vi "Calculate Total Ramp Period.vi"(0 "Start Delay In":dbl[](array[numeric]), 2 "Default Ramp Rate":bool[](array[boolean]), 5 "Relative To":T1[](array[typedef]) items=["Power sequence start", "Previous source start", "Previous source end"], 7 "Level":dbl[](array[numeric]), 9 "Ramp Rate":dbl[](array[numeric]), 11 "Sequence Delta":dbl[](array[numeric])) -> (4 "Accumulative Start delays":dbl[](array[numeric]), 6 "Total Power Seq Period":dbl format="%#_6p", 8 "Rising Period":dbl[](array[numeric]) format="%#_6p", 10 "Max Sequence Period Index":i32)   [LabVIEW 2024, in "devicePowerSequencerCoreLogic.lvlib"]
uses:
  devicePowerSequencerCoreLogic.lvlib
  controls/Relative To.ctl
  Device Power Sequencer.lvlib
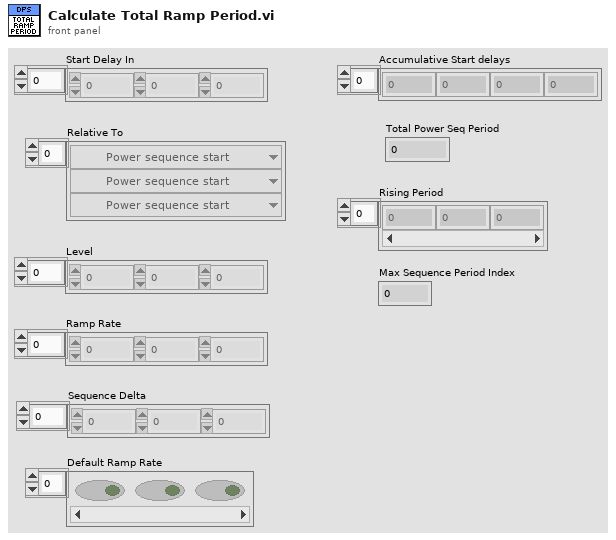
[diagram p1: front panel]
types:
  T1 = typedef "Device Power Sequencer.lvlib/Relative To.ctl" = u32
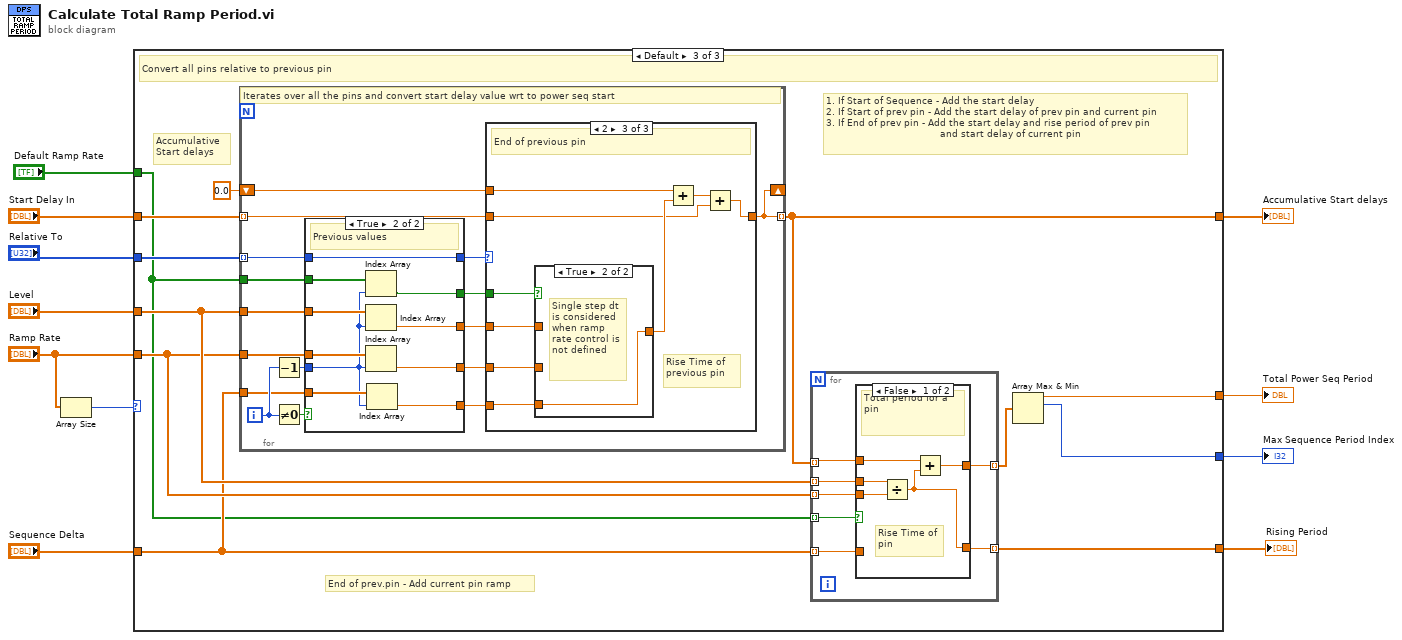
[diagram p0: block diagram]
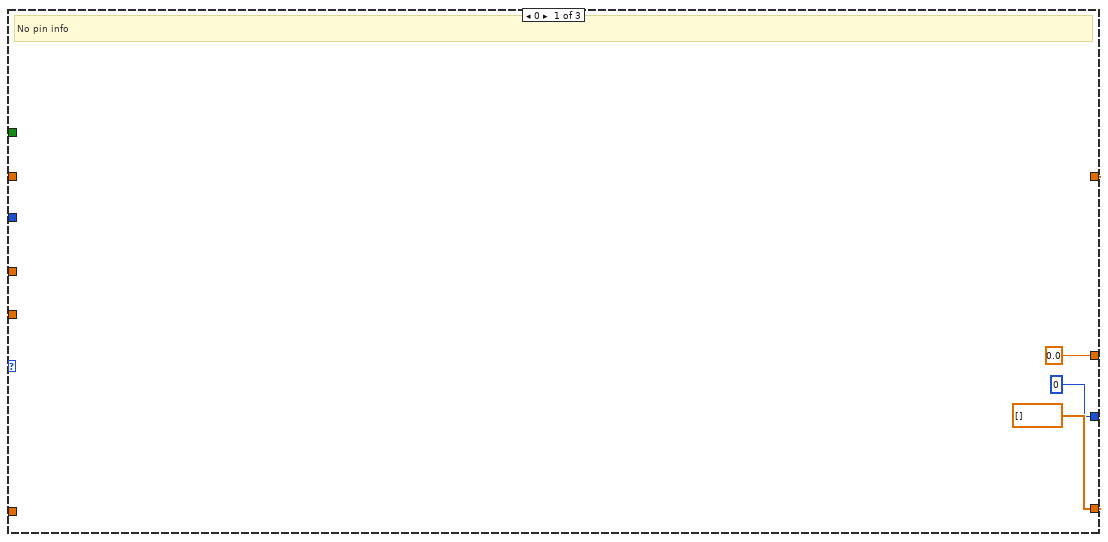
[diagram p2: hidden frame]
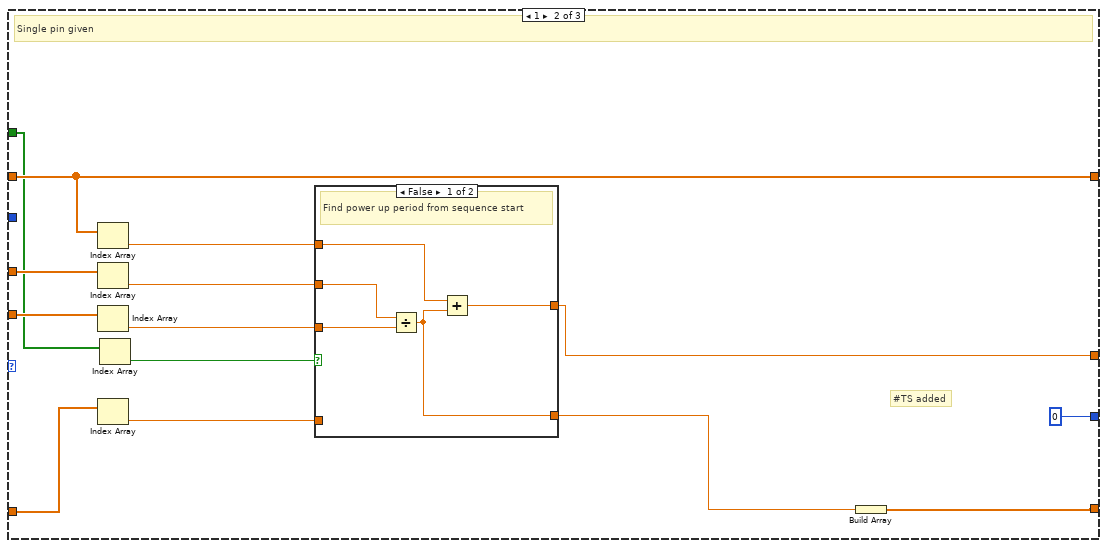
[diagram p3: hidden frame]
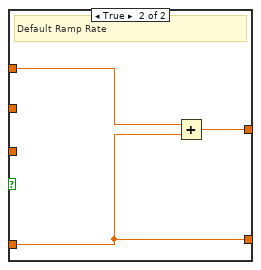
[diagram p4: hidden frame]
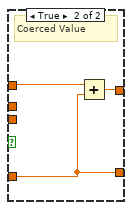
[diagram p5: hidden frame]
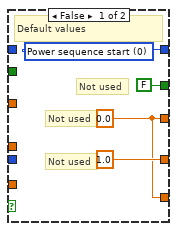
[diagram p6: hidden frame]
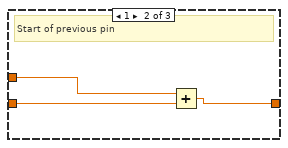
[diagram p8: hidden frame]
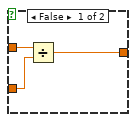
[diagram p9: hidden frame]
diagram:
  n1 = Array Size(array="Ramp Rate") -> (size(s)=w7:i32)
  n2 = case shown="Default" w7 {
    tunnel: "Start Delay In" -> [_ w21 w48]
    tunnel: "Relative To" -> [_ _ w47]
    tunnel: "Level" -> [_ w28 w45]
    tunnel: "Ramp Rate" -> [_ w27 w44]
    tunnel: [0.0 w20 w40] -> w9
    tunnel: [w14 w18 w39] -> w3
    tunnel: "Sequence Delta" -> [_ w23 w42]
    tunnel: [w14 w21 w41] -> w4
    tunnel: [0 0 w38] -> w2
    tunnel: "Default Ramp Rate" -> [_ w15 w37]
    frame 0 {
      w14 = dbl[] []
      # "No pin info"
    }
    frame 1 {
      # "#TS added"
      # "Single pin given"
      n3 = Index Array(array=w21) -> (element=w24:dbl)  [unwired: 1 in]
      n4 = Index Array(array=w28) -> (element=w25:dbl)  [unwired: 1 in]
      n5 = Index Array(array=w27) -> (element=w26:dbl)  [unwired: 1 in]
      n6 = Index Array(array=w23) -> (element=w22:dbl)  [unwired: 1 in]
      n7 = Index Array(array=w15) -> (element=w16:bool)  [unwired: 1 in]
      n8 = case shown="False" w16 {
        tunnel: [w33 w35] -> w20
        tunnel: w26 -> [w32 _]
        tunnel: w25 -> [w31 _]
        tunnel: w24 -> [w30 w36]
        tunnel: w22 -> [_ w34]
        tunnel: [w29 w34] -> w19
        frame False {
          # "Find power up period from sequence start"
          n9 = Divide(x=w31, y=w32) -> (x/y=w29:dbl)
          n10 = Add(x=w30, y=w29) -> (x+y=w33:dbl)
        }
        frame True {
          # "Default Ramp Rate"
          n11 = Add(x=w36, y=w34) -> (x+y=w35:dbl)
        }
      }
      n12 = Build Array(w19) -> (w18:dbl[])
    }
    frame Default {
      # "1. If Start of Sequence - Add the start delay\n2. If Start of prev pin - Add the start delay of prev pin and current pin\n3. If End of prev pin - Add the start delay and rise period of prev pin \n                                      and start delay of current pin"
      # "End of prev.pin - Add current pin ramp"
      # "Accumulative\nStart delays"
      # "Convert all pins relative to previous pin"
      n13 = for {
        tunnel: w48 -> [w79] mode=indexing
        tunnel: w47 -> [w67] mode=indexing
        tunnel: w44 -> [w75]
        tunnel: [w74] -> w41 mode=indexing
        shift-right: [w74] -> _
        shift-left: 0.0 ("Numeric") -> [w78]
        tunnel: w45 -> [w76]
        tunnel: w42 -> [w69]
        tunnel: w37 -> [w65]
        i -> [w73]
        # "Iterates over all the pins and convert start delay value wrt to power seq start"
        n14 = Decrement(x=w73) -> (x-1=w72:i32)
        n15 = Not Equal To 0?(x=w73) -> (x != 0?=w77:bool)
        n16 = case shown="True" w77 {
          tunnel: w76 -> [_ w93]
          tunnel: w75 -> [_ w92]
          tunnel: w72 -> [_ w85]
          tunnel: [w82 w91] -> w71
          tunnel: [1.0 ("Numeric") w90] -> w70
          tunnel: w69 -> [_ w89]
          tunnel: [w82 w88] -> w68
          tunnel: w67 -> [_ w87]
          tunnel: [w81 w87] -> w66
          tunnel: w65 -> [_ w86]
          tunnel: [FALSE ("Default Ramp Rate?") w84] -> w64
          frame False {
            w81 = T1 0 items=["Power sequence start", "Previous source start", "Previous source end"] ("Relative To")
            w82 = 0.0 ("Numeric")
            # "Not used"
            # "Not used"
            # "Not used"
            # "Default values"
          }
          frame True {
            # "Previous values"
            n17 = Index Array(array=w86, index=w85) -> (element=w84:bool)
            n18 = Index Array(array=w93, index=w85) -> (element=w91:dbl)
            n19 = Index Array(array=w92, index=w85) -> (element=w90:dbl)
            n20 = Index Array(array=w89, index=w85) -> (element=w88:dbl)
          }
        }
        n21 = case shown="2" w66 {
          tunnel: w79 -> [w94 w96 w102]
          tunnel: [w94 w95 w104] -> w74
          tunnel: w78 -> [_ w97 w105]
          tunnel: w71 -> [_ _ w101]
          tunnel: w70 -> [_ _ w99]
          tunnel: w68 -> [_ _ w100]
          tunnel: w64 -> [_ _ w98]
          frame 0, Default {
            # "Start of sequence"
          }
          frame 1 {
            # "Start of previous pin"
            n22 = Add(x=w97, y=w96) -> (x+y=w95:dbl)
          }
          frame 2 {
            # "Rise Time of previous pin"
            # "End of previous pin"
            n23 = case shown="True" w98 {
              tunnel: [w109 w110] -> w103
              tunnel: w101 -> [w108 _]
              tunnel: w99 -> [w107 _]
              tunnel: w100 -> [_ w110]
              frame False {
                n24 = Divide(x=w108, y=w107) -> (x/y=w109:dbl)
              }
              frame True {
                # "Single step dt is considered when ramp rate control is not defined"
              }
            }
            n25 = Add(x=w105, y=w103) -> (x+y=w106:dbl)
            n26 = Add(x=w106, y=w102) -> (x+y=w104:dbl)
          }
        }
      }
      n27 = for {
        tunnel: w45 -> [w55] mode=indexing
        tunnel: w44 -> [w52] mode=indexing
        tunnel: w41 -> [w54] mode=indexing
        tunnel: [w53] -> w43 mode=indexing
        tunnel: w42 -> [w51] mode=indexing
        tunnel: [w50] -> w39 mode=indexing
        tunnel: w37 -> [w49] mode=indexing
        n28 = case shown="False" w49 {
          tunnel: w55 -> [w60 _]
          tunnel: w52 -> [w59 _]
          tunnel: w54 -> [w58 w63]
          tunnel: [w57 w62] -> w53
          tunnel: w51 -> [_ w61]
          tunnel: [w56 w61] -> w50
          frame False {
            # "Rise Time of pin"
            # "Total period for a pin"
            n29 = Divide(x=w60, y=w59) -> (x/y=w56:dbl)
            n30 = Add(x=w58, y=w56) -> (x+y=w57:dbl)
          }
          frame True {
            # "Coerced Value"
            n31 = Add(x=w63, y=w61) -> (x+y=w62:dbl)
          }
        }
      }
      n32 = Array Max & Min(array=w43) -> (max value=w40:dbl, max index (indices)=w38:i32)  [unwired: 2 out]
    }
  }
  "Total Power Seq Period" <- w9
  "Rising Period" <- w3
  "Accumulative Start delays" <- w4
  "Max Sequence Period Index" <- w2
